vi "TwH5SetMassCalib.vi"(0 "error in (no error)":errorcluster, 5 "mode":i32, 7 "nbrParams":i32, 9 "p":dbl[](array[numeric]), 11 "nbrPoints":i32, 12 "mass":dbl[](array[numeric]), 13 "tof":dbl[](array[numeric]), 14 "weight":dbl[](array[numeric])) -> (4 "error out":errorcluster)   [LabVIEW 2009]
uses:
  TwH5Dll.dll
panel:
  in  "filename":string
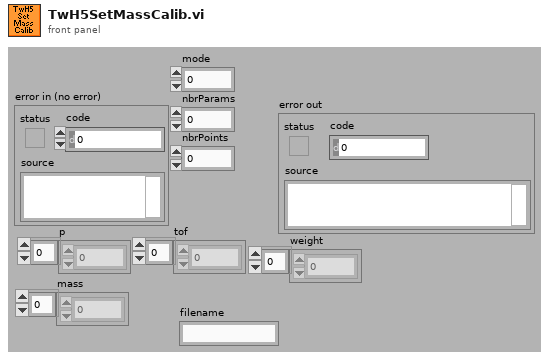
[diagram p1: front panel]
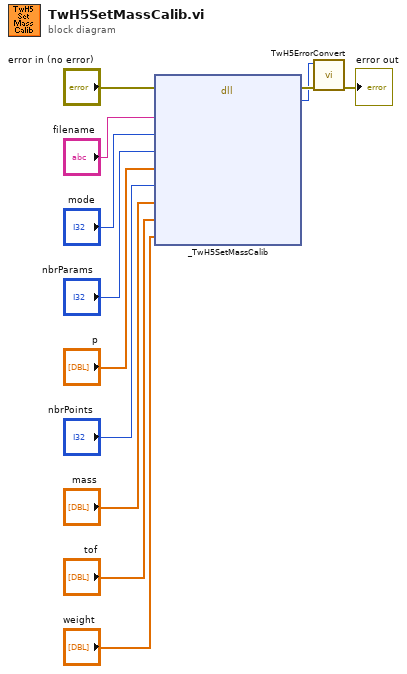
[diagram p0: block diagram]
diagram:
  n1 = dll-call lib="C:/src/85_TofDaq_current/DllWrappers/LabView/TwH5Dll/TwH5Dll.dll" fn="_TwH5SetMassCalib"(error in="error in (no error)", "filename"="filename", "mode"="mode", "nbrParams"="nbrParams", "p"="p", "nbrPoints"="nbrPoints", "mass"="mass", "tof"="tof", "weight"="weight") -> (error out=w11:errorcluster, "TwRetVal"=w10:i32)  [unwired: 10 in, 1 out]
  n2 = call "TwH5ErrorConvert.vi"("error in (no error)"=w11, "error code"=w10) -> ("error out"=→"error out":errorcluster)  [unwired: 9 out]
